vi "Teleop Pike Control.vi"(8 "Manipulator D-Pad":T1, 9 "Manipulator Buttons":T2, 10 "Driver D-Pad":T1, 11 "Driver Buttons":T2) -> ()   [LabVIEW 2014]
uses:
  Real-Life Controls/Button Cluster.ctl
  Real-Life Controls/D-Pad.ctl
  Pike Command.ctl
  Pike Mode.ctl
  Common Code/Change Detect Boolean.vi
  Robot Global Data.vi
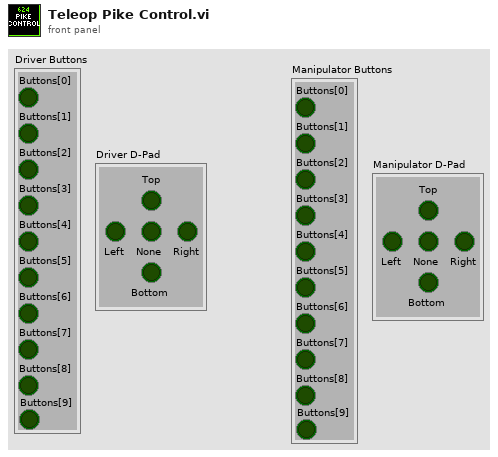
[diagram p1: front panel]
types:
  T1 = typedef "D-Pad.ctl" = cluster{"Top":bool, "Bottom":bool, "None":bool, "Right":bool, "Left":bool}
  T2 = typedef "Button Cluster.ctl" = cluster{"Buttons[0]":bool, "Buttons[1]":bool, "Buttons[2]":bool, "Buttons[3]":bool, "Buttons[4]":bool, "Buttons[5]":bool, "Buttons[6]":bool, "Buttons[7]":bool, "Buttons[8]":bool, "Buttons[9]":bool}
  T3 = typedef "Pike Mode.ctl" = enum16{"Idle", "Auto Down", "Auto Up", "Manual Down", "Manual Up"}
  T4 = typedef "Pike Command.ctl" = cluster{"Command":T3}
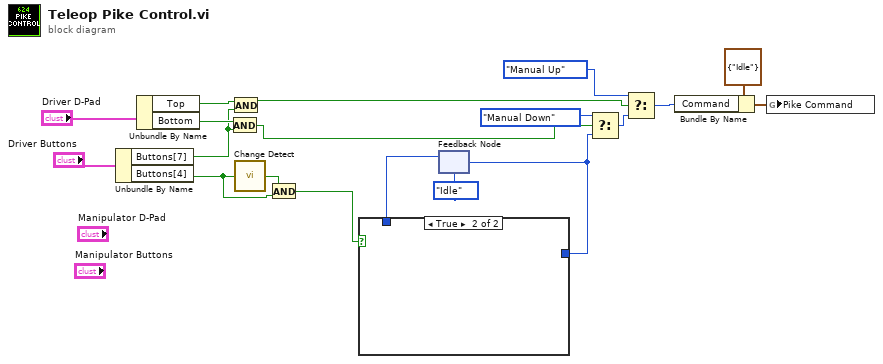
[diagram p0: block diagram]
diagram:
  n1 = Unbundle By Name("Driver Buttons") -> ("Buttons[7]"=w15:bool, "Buttons[4]"=w5:bool)
  n2 = Unbundle By Name("Driver D-Pad") -> ("Top"=w17:bool, "Bottom"=w16:bool)
  n3 = And(x=w16, y=w15) -> (x .and. y?=w8:bool)
  n4 = And(x=w17, y=w15) -> (x .and. y?=w12:bool)
  n5 = call-poly "Change Detect.vi"("In"=w5) -> ("Changed?"=w6:bool)
  n6 = And(x=w6, y=w5) -> (x .and. y?=w1:bool)
  n7 = feedback #1(Pike_Mode."Idle" ("Command")) -> (w4:T3)
  n8 = case shown="True" w1 {
    tunnel: w4 -> [w20 _]
    tunnel: [w20 _] -> w2
    frame False {
    }
    frame True {
    }
  }
  n9 = feedback-in #1(w2) -> ()
  n10 = Select(t=Pike_Mode."Manual Down" ("Command"), s=w8, f=w2) -> (s? t:f=w10:T3)
  n11 = Select(t=Pike_Mode."Manual Up" ("Command"), s=w12, f=w10) -> (s? t:f=w7:T3)
  n12 = Bundle By Name(cluster=T4 {"Command"=enum."Idle"} ("Pike Command"), "Command"=w7) -> (w13:T4)
  n13 = global write "Robot Global Data.vi" "Pike Command"(w13) -> ()
